vi "move item between listboxes.vi"(8 "error in":errorcluster, 10 "target":refnum<vi>, 11 "source":refnum<vi>) -> (0 "error out":errorcluster, 2 "new target":string[](array[string]), 3 "new source":string[](array[string]))   [LabVIEW 2014, in "SequencerActionScript.lvclass"]
doc: "NI Tag Bus Module Framework 1.0.2.36\nNI Systems Engineering"
uses:
  SequencerActionScript.lvclass
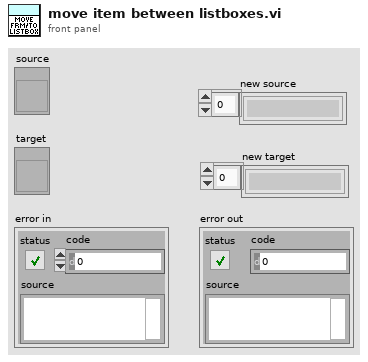
[diagram p1: front panel]
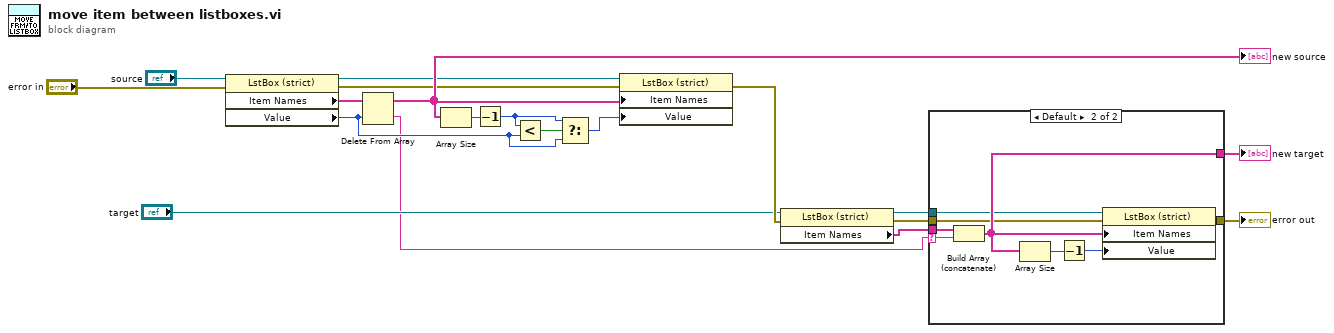
[diagram p0: block diagram]
diagram:
  n1 = property class="LstBox (strict)"(reference="source", error in="error in") -> (reference out=w4:refnum<vi>, error out=w3:errorcluster, "Item Names"=w2:string[], "Value"=w8:i32)
  n2 = Delete From Array(array=w2, index=w8) -> (deleted portion=w1:string, array with subset deleted=w5:string[])  [unwired: 1 in]
  "new source" <- w5
  n3 = Array Size(array=w5) -> (size(s)=w6:i32)
  n4 = Decrement(x=w6) -> (x-1=w9:i32)
  n5 = Less?(x=w9, y=w8) -> (x < y?=w7:bool)
  n6 = Select(t=w9, s=w7, f=w8) -> (s? t:f=w10:i32)
  n7 = property class="LstBox (strict)"(reference=w4, error in=w3, "Item Names"=w5, "Value"=w10) -> (error out=w15:errorcluster)  [unwired: 1 out]
  n8 = property class="LstBox (strict)"(reference="target", error in=w15) -> (reference out=w12:refnum<vi>, error out=w13:errorcluster, "Item Names"=w18:string[])
  n9 = case shown="Default" w1 {
    selector: w1 -> [_ w22]
    tunnel: [w20 w27] -> w19
    tunnel: w18 -> [w20 w26]
    tunnel: [w21 w25] -> w17
    tunnel: w13 -> [w21 w24]
    tunnel: w12 -> [_ w23]
    frame "" {
    }
    frame Default {
      n10 = Build Array (concatenate)(w26, w22) -> (w27:string[])
      n11 = Array Size(array=w27) -> (size(s)=w29:i32)
      n12 = Decrement(x=w29) -> (x-1=w28:i32)
      n13 = property class="LstBox (strict)"(reference=w23, error in=w24, "Item Names"=w27, "Value"=w28) -> (error out=w25:errorcluster)  [unwired: 1 out]
    }
  }
  "error out" <- w17
  "new target" <- w19
